vi "Exercise6_2.vi"() -> ()   [LabVIEW 2015]
doc: "This VI demonstrates how the order in which you apply transformations to an object in a 3D scene affects the object's position and orientation within the scene. \n\n<b>Rotate then Translate:</b>\nIf you apply a rotation to an object as the first transformation, the object rotates around its parent's axis, which exists in spatially the same place as the object's own axis. Regardless of what transformations follow the rotation, the object appears to rotate around its own axis. If you apply a translation after the rotation, the object appears offset from its parent and still spinning around its own axis.\n\n<b>Translate then Rotate:</b>\nIf you apply a translation to an object as the first transformation, the object still appears offset from its parent. However, if you then apply a rotation to the object, the object rotates around its parent by the angle you specify with the Translate Object VI."
uses:
  <vilib>/Analysis/Matrix/Datatypes/RealMatrix.ctl
  <vilib>/Analysis/Matrix/NI_Matrix.lvlib
panel:
  in  "RPY angles":cluster{"roll":dbl, "pitch":dbl, "yaw":dbl}
  out "noa":cluster{T1, T1, T1}
  out "error out":errorcluster
  out "Euler angles":T2
  out "Orientation matrix":dbl[][](array[numeric])
  in  "XYZ":dbl[](array[numeric]) format="%0.2f"
  in  "Stop":bool
  out "3D Picture":refnum<vi>(3d-picture)
  # "Position and Orientation POSE"
  # "XYZ --> Mobile frame\nZYX --> Fixed frame"
  # "Com a l'exercici 5, en lloc de zeros hi ha zeros numèrics.\nNo he trobat com canviar-ho, però el resultat és correcte\nde tota manera."
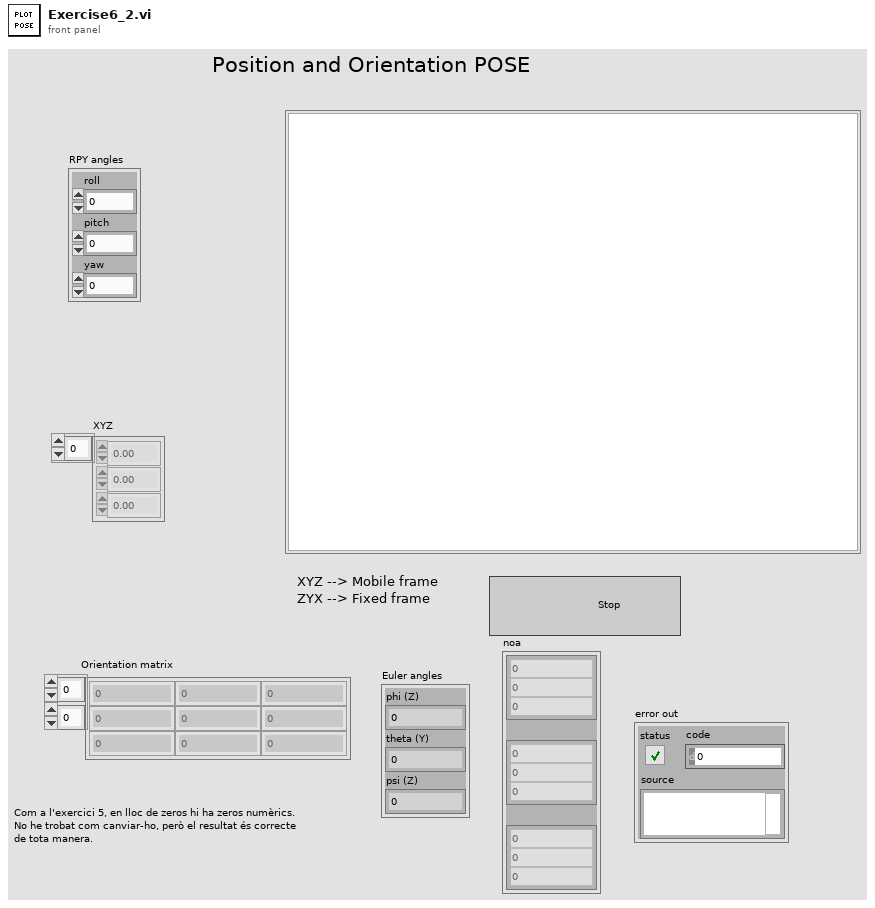
[diagram p1: front panel]
types:
  T1 = typedef "NI_Matrix.lvlib/RealMatrix.ctl" = dbl[][]
  T2 = cluster{"phi (Z)":dbl, "theta (Y)":dbl, "psi (Z)":dbl}
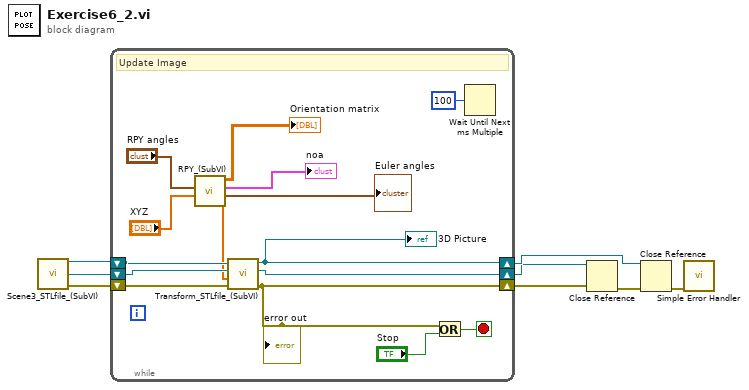
[diagram p0: block diagram]
diagram:
  n1 = call "Scene3_STLfile_(SubVI).vi"() -> ("error out"=w1:errorcluster, "New Object Out"=w2:refnum<vi>, "SceneObject out"=w3:refnum<vi>)  [unwired: 9 in]
  n2 = while {
    shift-right: [w15] -> w7
    shift-left: w1 -> [w18]
    shift-right: [w16] -> w4
    shift-left: w2 -> [w19]
    shift-right: [w17] -> w8
    shift-left: w3 -> [w20]
    stop <- w22 stop-if-true
    # "Update Image"
    n3 = call "RPY_(SubVI).vi"("XYZ"="XYZ", "RPY angles"="RPY angles") -> ("POSE"=w14:dbl[], "Euler angles"=→"Euler angles":T2, "noa"=→"noa":cluster{T1, T1, T1}, "Rotation matrix"=→"Orientation matrix":dbl[][])  [unwired: 6 in]
    n4 = call "Transform_STLfile_(SubVI).vi"("error in (no error)"=w18, "POSE"=w14, "New Object In"=w19, "SceneObject In"=w20) -> ("error out"=w15:errorcluster, "New Object out"=w16:refnum<vi>, "SceneObject Out"=w17:refnum<vi>)  [unwired: 5 in]
    "3D Picture" <- w17
    "error out" <- w15
    n5 = Or(x=w15, y="Stop") -> (x .or. y?=w22:bool)
    n6 = Wait Until Next ms Multiple(millisecond multiple=u32 100 ("milliseconds to wait")) -> ()  [unwired: 1 out]
  }
  n7 = Close Reference(reference=w4, error in (no error)=w7) -> (error out=w5:errorcluster)
  n8 = Close Reference(reference=w8, error in (no error)=w5) -> (error out=w6:errorcluster)
  n9 = call <vilib>:"Simple Error Handler.vi"("error in (no error)"=w6) -> ()  [unwired: 4 in, 5 out]
